vi "InstruDataRead_DP_ver2.1.vi"(8 "error in":errorcluster, 9 "memory of # of pts in buffer":i32[](array[numeric]), 10 "Const I output":dbl[](array[numeric]), 11 "output cluster":T1={"Main Sweep"=0, "Steps Config:"={"total points:"=0, "Step Delay (s)"=0.0, "Ini Delay (s)"=0.0, "# of steps:"=0}, "Temperature Control (ITC 503):"={"GPIB ADR"=0, "Change Heater?"={"Heater?"=FALSE, "Heater"=0}, "Change Temp?"={"Change T?"=FALSE, "Set T (K)"=0.0}, "Cluster"={"Heat Auto?"=FALSE, "Manual Heat?"=FALSE, "Heater (%)"=0.0}, "Change PID?"={"Change PID?"=FALSE, "P"=0.0, "I"=0.0, "D"=0.0}, "Change Para?"=FALSE, "Sensor"=1}, "Temperature Control (LS 340):"={"GPIB ADR"=0, "From (K)"=0.0, "To (K)"=0.0, "Rate (K/min)"=0.0, "Delta T (0.08K)"=0.0, "Temp. Header"="", "T Display Control"={"Ch B"=FALSE, "Ch C"=FALSE, "Ch D"=FALSE}}, "Magnet Control (IPS 120-10)"={"Action"=0, "Standby (s)"=0.0, "Heater on (s)"=0.0, "Sweep Setup "=[], "GPIB ADR"=0, "Change Para?"=FALSE}, "Keithley 6221 :"=[], "Measuring Instruments : "=[], "Lock-In SR7265 :"=[], "Deascription of \nthis measurement"="", "Instruments Config:"=[], "LS372 Bridge : 2"=[{"GPIB"=0, "Excitation"=0, "Autorange?"=FALSE, "Range"=0, "Current"=0, "Voltage"=0, "DataHeader"="Rx;Ry"}], "Magnet Control (CS4) 2"={"Action"=1, "Standby (s)"=0.0, "Heater on (s)"=300.0, "Sweep Setup "=[], "GPIB ADR"=0, "Change Para?"=FALSE}} {"Magnet Control (CS4) 2"."GPIB ADR" items=["None"=0, "25"=25]; "Magnet Control (CS4) 2"."Sweep Setup"."Rate in Range (T/min)" min=0.001 max=0.5 step=0.001; "Magnet Control (CS4) 2"."Sweep Setup"."Hold(min)" min=0.0; "Magnet Control (CS4) 2"."Sweep Setup"."Set Point (T)" min=-9.0 max=9.0 step=0.001; "Magnet Control (CS4) 2"."Action" items=["Up", "Down", "Pause", "Zero"]; "LS372 Bridge : 2"."Voltage" items=["2.00 uV"=1, "6.32 uV"=2, "20.0 uV"=3, "63.2 uV"=4, "200 uV"=5, "632 uV"=6, "2.0 mV"=7, "6.32 mV"=8]; "LS372 Bridge : 2"."Current" items=["1.00 pA"=1, "3.16 pA"=2, "10.0 pA"=3, "31.6 pA"=4, "100 pA"=5, "316 pA"=6, "1.00 nA"=7, "3.16 nA"=8, "10 nA"=9, "31.6 nA"=10, "100 nA"=11, "316 nA"=12, "1.00 uA"=13, "3.16 uA"=14, "10.0 uA"=15, "31.6 uA"=16, "100 uA"=17, "316 uA"=18, "1.00 mA"=19, "3.16 mA"=20, "10.0 mA"=21, "31.6 mA"=22]; "LS372 Bridge : 2"."Range" items=["2.0 m"=1, "6.32 m"=2, "20.0 m"=3, "63.2 m"=4, "200 m"=5, "632 m"=6, "2.00"=7, "6.32"=8, "20.0"=9, "63.2"=10, "200"=11, "632"=12, "2.00 k"=13, "6.32 k"=14, "20.0 k"=15, "63.2 k"=16, "200 k"=17, "632 k"=18, "2.00 M"=19, "6.32 M"=20, "20.0 M"=21, "63.2 M"=22]; "LS372 Bridge : 2"."Excitation" items=["Voltage", "Current"]; "LS372 Bridge : 2"."GPIB" items=["None"=0, "9"=9]; "Main Sweep" items=["Time", "DC Current", "Delta Current", "Pulse Delta Current", "Sine Current", "Lock-in Vosc"]; "Temperature Control (ITC 503):"."Sensor" items=["T2", "T3"]; "Magnet Control (IPS 120-10)"."Action" items=["Hold", "To Set point", "To Zero", "Clamp"]; "Keithley 6221 :"."Sweep Mode" items=["Linear", "Log", "Exp", "Inverse", "Manual"]}) -> (0 "error out":errorcluster, 1 "memory of # of pts in buffer update":i32[](array[numeric]), 2 "Data":dbl[](array[numeric]), 3 "output cluster 2":T1={"Main Sweep"=0, "Steps Config:"={"total points:"=0, "Step Delay (s)"=0.0, "Ini Delay (s)"=0.0, "# of steps:"=0}, "Temperature Control (ITC 503):"={"GPIB ADR"=0, "Change Heater?"={"Heater?"=FALSE, "Heater"=0}, "Change Temp?"={"Change T?"=FALSE, "Set T (K)"=0.0}, "Cluster"={"Heat Auto?"=FALSE, "Manual Heat?"=FALSE, "Heater (%)"=0.0}, "Change PID?"={"Change PID?"=FALSE, "P"=0.0, "I"=0.0, "D"=0.0}, "Change Para?"=FALSE, "Sensor"=1}, "Temperature Control (LS 340):"={"GPIB ADR"=0, "From (K)"=0.0, "To (K)"=0.0, "Rate (K/min)"=0.0, "Delta T (0.08K)"=0.0, "Temp. Header"="", "T Display Control"={"Ch B"=FALSE, "Ch C"=FALSE, "Ch D"=FALSE}}, "Magnet Control (IPS 120-10)"={"Action"=0, "Standby (s)"=0.0, "Heater on (s)"=0.0, "Sweep Setup "=[], "GPIB ADR"=0, "Change Para?"=FALSE}, "Keithley 6221 :"=[], "Measuring Instruments : "=[], "Lock-In SR7265 :"=[], "Deascription of \nthis measurement"="", "Instruments Config:"=[], "LS372 Bridge : 2"=[{"GPIB"=0, "Excitation"=0, "Autorange?"=FALSE, "Range"=0, "Current"=0, "Voltage"=0, "DataHeader"="Rx;Ry"}], "Magnet Control (CS4) 2"={"Action"=1, "Standby (s)"=0.0, "Heater on (s)"=300.0, "Sweep Setup "=[], "GPIB ADR"=0, "Change Para?"=FALSE}} {"Magnet Control (CS4) 2"."GPIB ADR" items=["None"=0, "25"=25]; "Magnet Control (CS4) 2"."Sweep Setup"."Rate in Range (T/min)" min=0.001 max=0.5 step=0.001; "Magnet Control (CS4) 2"."Sweep Setup"."Hold(min)" min=0.0; "Magnet Control (CS4) 2"."Sweep Setup"."Set Point (T)" min=-9.0 max=9.0 step=0.001; "Magnet Control (CS4) 2"."Action" items=["Up", "Down", "Pause", "Zero"]; "LS372 Bridge : 2"."Voltage" items=["2.00 uV"=1, "6.32 uV"=2, "20.0 uV"=3, "63.2 uV"=4, "200 uV"=5, "632 uV"=6, "2.0 mV"=7, "6.32 mV"=8]; "LS372 Bridge : 2"."Current" items=["1.00 pA"=1, "3.16 pA"=2, "10.0 pA"=3, "31.6 pA"=4, "100 pA"=5, "316 pA"=6, "1.00 nA"=7, "3.16 nA"=8, "10 nA"=9, "31.6 nA"=10, "100 nA"=11, "316 nA"=12, "1.00 uA"=13, "3.16 uA"=14, "10.0 uA"=15, "31.6 uA"=16, "100 uA"=17, "316 uA"=18, "1.00 mA"=19, "3.16 mA"=20, "10.0 mA"=21, "31.6 mA"=22]; "LS372 Bridge : 2"."Range" items=["2.0 m"=1, "6.32 m"=2, "20.0 m"=3, "63.2 m"=4, "200 m"=5, "632 m"=6, "2.00"=7, "6.32"=8, "20.0"=9, "63.2"=10, "200"=11, "632"=12, "2.00 k"=13, "6.32 k"=14, "20.0 k"=15, "63.2 k"=16, "200 k"=17, "632 k"=18, "2.00 M"=19, "6.32 M"=20, "20.0 M"=21, "63.2 M"=22]; "LS372 Bridge : 2"."Excitation" items=["Voltage", "Current"]; "LS372 Bridge : 2"."GPIB" items=["None"=0, "9"=9]; "Main Sweep" items=["Time", "DC Current", "Delta Current", "Pulse Delta Current", "Sine Current", "Lock-in Vosc"]; "Temperature Control (ITC 503):"."Sensor" items=["T2", "T3"]; "Magnet Control (IPS 120-10)"."Action" items=["Hold", "To Set point", "To Zero", "Clamp"]; "Keithley 6221 :"."Sweep Mode" items=["Linear", "Log", "Exp", "Inverse", "Manual"]}, 4 "B (T)":string, 5 "T2 (K)":string, 6 "T3 (K)":string, 7 "T1 (K)":string)   [LabVIEW 2012]
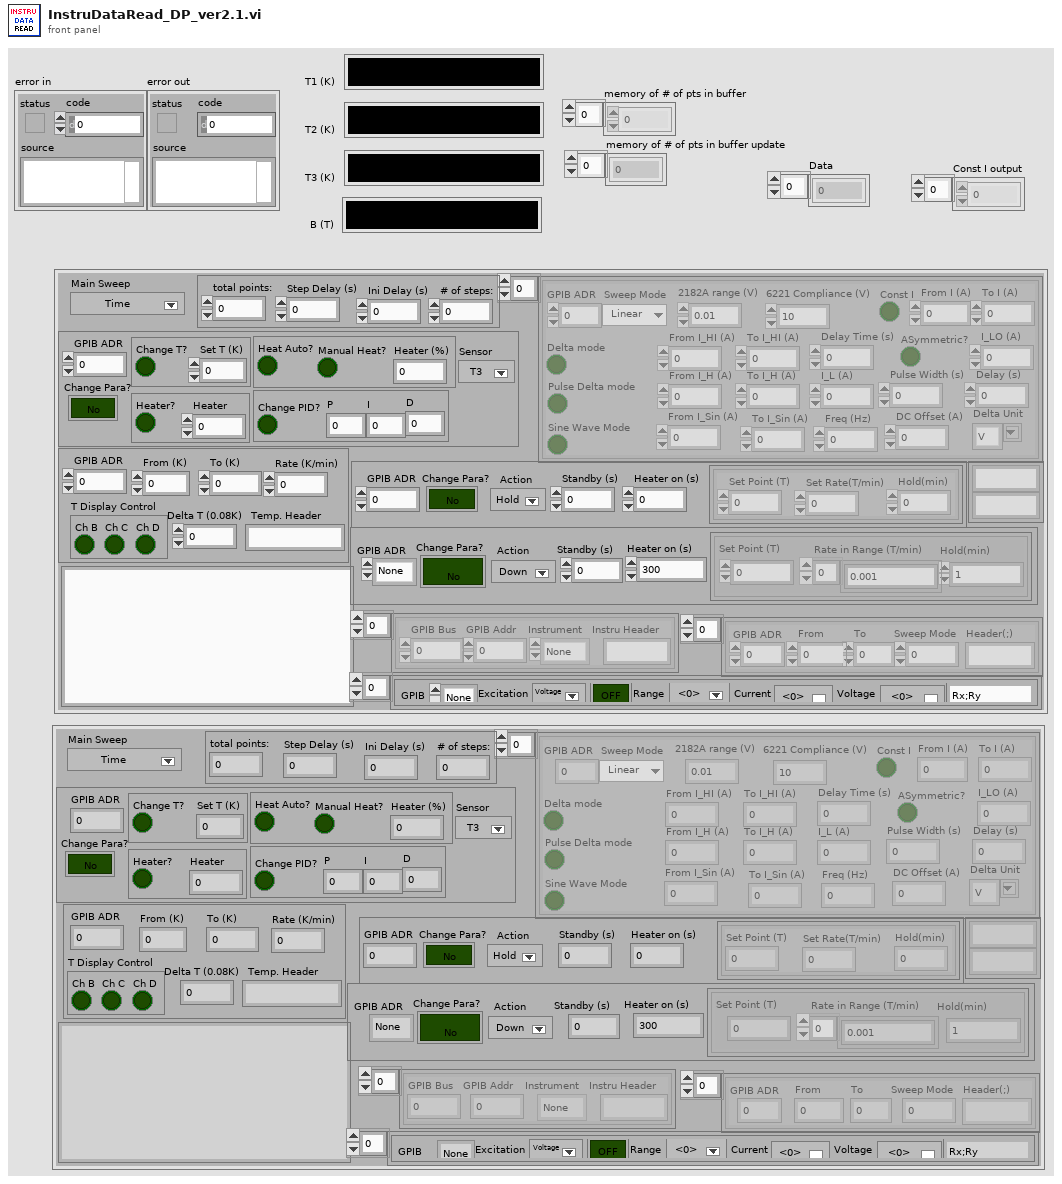
[diagram p1: front panel]
types:
  T1 = cluster{"Main Sweep":u8, "Steps Config:":cluster{"total points:":u32, "Step Delay (s)":dbl, "Ini Delay (s)":dbl, "# of steps:":u32}, "Temperature Control (ITC 503):":cluster{"GPIB ADR":u16, "Change Heater?":cluster{"Heater?":bool, "Heater":u8}, "Change Temp?":cluster{"Change T?":bool, "Set T (K)":dbl}, "Cluster":cluster{"Heat Auto?":bool, "Manual Heat?":bool, "Heater (%)":dbl}, "Change PID?":cluster{"Change PID?":bool, "P":dbl, "I":dbl, "D":dbl}, "Change Para?":bool, "Sensor":u16}, "Temperature Control (LS 340):":cluster{"GPIB ADR":u16, "From (K)":dbl, "To (K)":dbl, "Rate (K/min)":dbl, "Delta T (0.08K)":dbl, "Temp. Header":string, "T Display Control":cluster{"Ch B":bool, "Ch C":bool, "Ch D":bool}}, "Magnet Control (IPS 120-10)":cluster{"Action":u16, "Standby (s)":dbl, "Heater on (s)":dbl, "Sweep Setup ":cluster{"Set Point (T)":dbl, "Set Rate(T/min)":dbl, "Hold(min)":dbl}[], "GPIB ADR":u16, "Change Para?":bool}, "Keithley 6221 :":cluster{"Delta mode":bool, "Const I":bool, "Pulse Delta mode":bool, "Sine Wave Mode":bool, "From I_HI (A)":dbl, "From I (A)":dbl, "I_LO (A)":dbl, "From I_H (A)":dbl, "I_L (A)":dbl, "Freq (Hz)":dbl, "From I_Sin (A)":dbl, "DC Offset (A)":dbl, "Delay Time (s)":dbl, "Pulse Width (s)":dbl, "Delay (s)":dbl, "To I (A)":dbl, "ASymmetric?":bool, "To I_HI (A)":dbl, "To I_H (A)":dbl, "To I_Sin (A)":dbl, "GPIB ADR":u16, "Sweep Mode":u8, "Delta Unit":string, "2182A range (V)":dbl, "6221 Compliance (V)":dbl}[], "Measuring Instruments : ":cluster{"GPIB Bus":dbl, "GPIB Addr":dbl, "Instrument":enum16{"None", "HP34401DMM", "Lockin 7265", "HP3456/7A", "HP3478A", "HP3325FG", "Keithley2182A"}, "Instru Header":string}[], "Lock-In SR7265 :":cluster{"GPIB ADR":u16, "From":dbl, "To":dbl, "Header(;)":string, "Sweep Mode":u8}[], "Deascription of \nthis measurement":string, "Instruments Config:":string[][], "LS372 Bridge : 2":cluster{"GPIB":u16, "Excitation":u16, "Autorange?":bool, "Range":u16, "Current":u16, "Voltage":u16, "DataHeader":string}[], "Magnet Control (CS4) 2":cluster{"Action":u16, "Standby (s)":dbl, "Heater on (s)":dbl, "Sweep Setup ":cluster{"Set Point (T)":dbl, "Hold(min)":dbl, "Rate in Range (T/min)":dbl[]}[], "GPIB ADR":u16, "Change Para?":bool}}
  T2 = cluster{"GPIB":u16, "Excitation":u16, "Autorange?":bool, "Range":u16, "Current":u16, "Voltage":u16, "DataHeader":string}[]
  T3 = cluster{"Delta mode":bool, "Const I":bool, "Pulse Delta mode":bool, "Sine Wave Mode":bool, "From I_HI (A)":dbl, "From I (A)":dbl, "I_LO (A)":dbl, "From I_H (A)":dbl, "I_L (A)":dbl, "Freq (Hz)":dbl, "From I_Sin (A)":dbl, "DC Offset (A)":dbl, "Delay Time (s)":dbl, "Pulse Width (s)":dbl, "Delay (s)":dbl, "To I (A)":dbl, "ASymmetric?":bool, "To I_HI (A)":dbl, "To I_H (A)":dbl, "To I_Sin (A)":dbl, "GPIB ADR":u16, "Sweep Mode":u8, "Delta Unit":string, "2182A range (V)":dbl, "6221 Compliance (V)":dbl}[]
  T4 = cluster{"GPIB Bus":dbl, "GPIB Addr":dbl, "Instrument":enum16{"None", "HP34401DMM", "Lockin 7265", "HP3456/7A", "HP3478A", "HP3325FG", "Keithley2182A"}, "Instru Header":string}[]
  T5 = cluster{"GPIB ADR":u16, "From":dbl, "To":dbl, "Header(;)":string, "Sweep Mode":u8}[]
  T6 = enum16{"None", "HP34401DMM", "Lockin 7265", "HP3456/7A", "HP3478A", "HP3325FG"}
  T7 = enum16{"None", "HP34401DMM", "Lockin 7265", "HP3456/7A", "HP3478A", "HP3325FG", "Keithley2182A"}
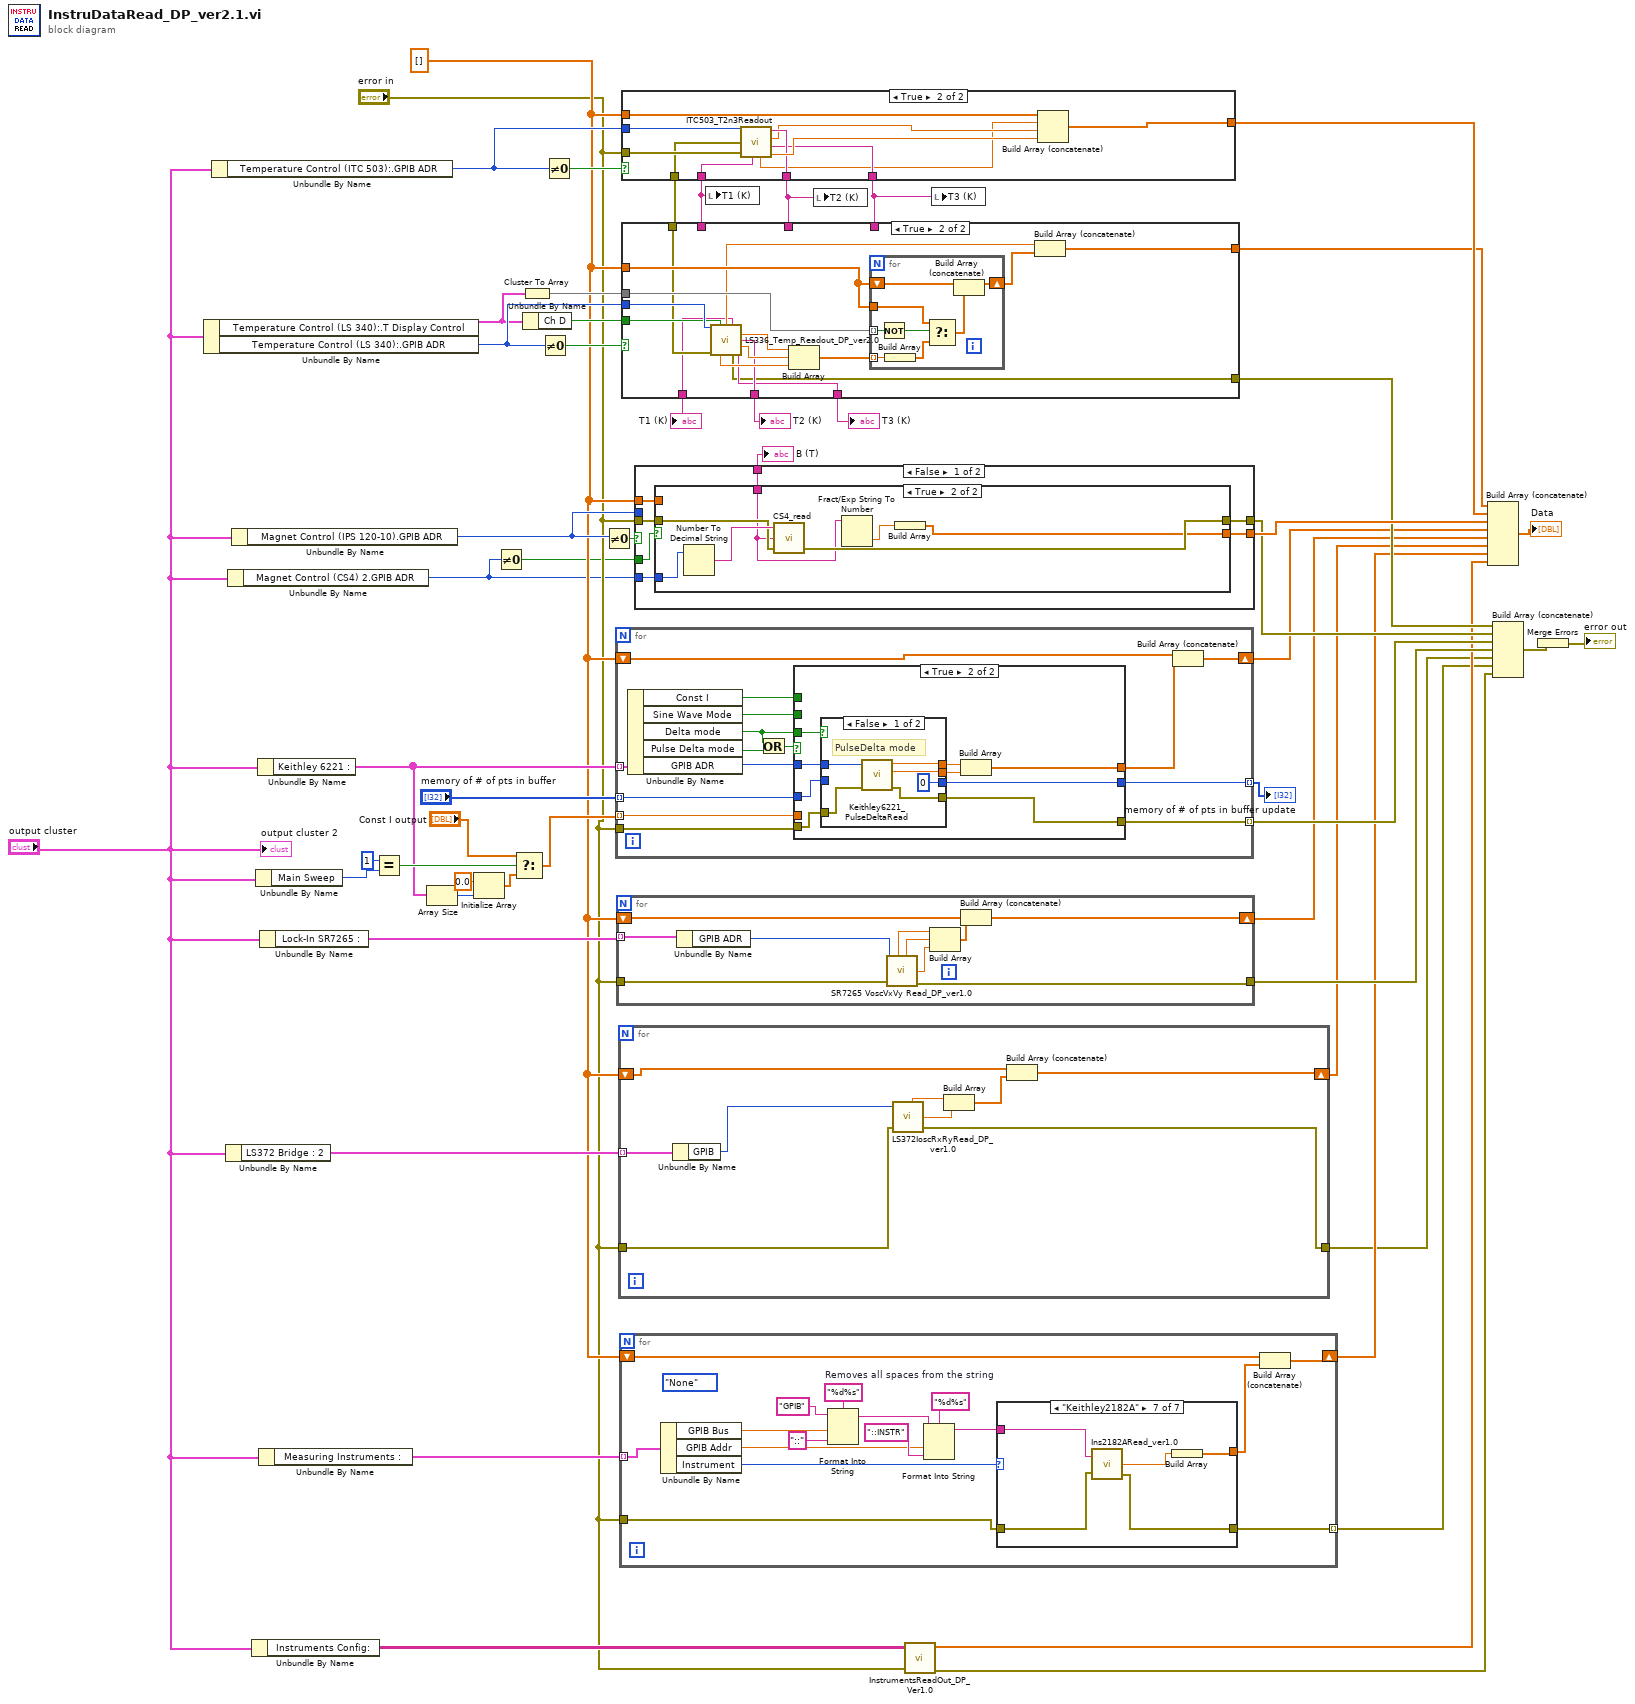
[diagram p0: block diagram]
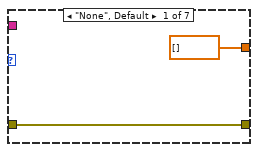
[diagram p2: hidden frame]
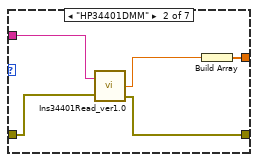
[diagram p3: hidden frame]
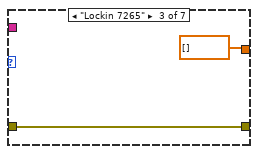
[diagram p4: hidden frame]
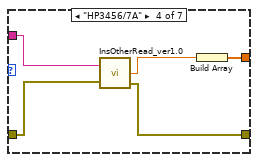
[diagram p5: hidden frame]
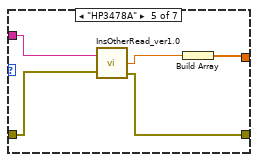
[diagram p6: hidden frame]
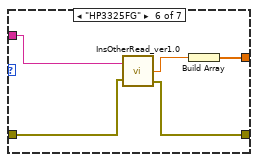
[diagram p7: hidden frame]
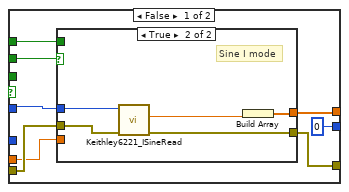
[diagram p8: hidden frame]
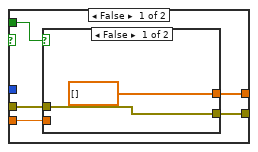
[diagram p9: hidden frame]
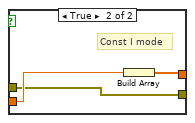
[diagram p10: hidden frame]
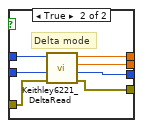
[diagram p11: hidden frame]
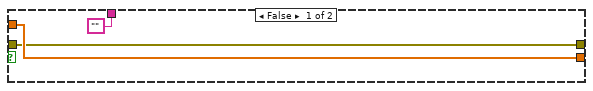
[diagram p12: hidden frame]
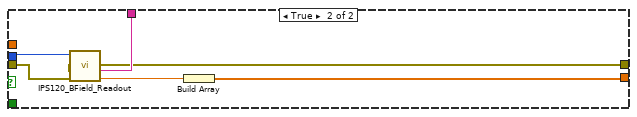
[diagram p13: hidden frame]
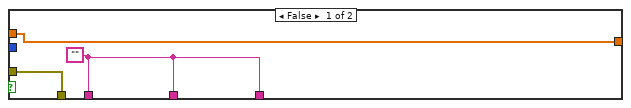
[diagram p14: hidden frame]
diagram:
  w7 = dbl[] []
  n1 = Unbundle By Name("output cluster") -> ("Temperature Control (LS 340):.T Display Control"=w52:cluster{"Ch B":bool, "Ch C":bool, "Ch D":bool}, "Temperature Control (LS 340):.GPIB ADR"=w54:u16)
  n2 = Unbundle By Name("output cluster") -> ("Temperature Control (ITC 503):.GPIB ADR"=w46:u16)
  n3 = Unbundle By Name("output cluster") -> ("LS372 Bridge : 2"=w8:T2)
  n4 = Unbundle By Name("output cluster") -> ("Magnet Control (CS4) 2.GPIB ADR"=w2:u16)
  n5 = Unbundle By Name("output cluster") -> ("Magnet Control (IPS 120-10).GPIB ADR"=w38:u16)
  n6 = Unbundle By Name("output cluster") -> ("Instruments Config:"=w26:string[][])
  n7 = Unbundle By Name("output cluster") -> ("Main Sweep"=w17:u8)
  n8 = Unbundle By Name("output cluster") -> ("Keithley 6221 :"=w12:T3)
  n9 = Unbundle By Name("output cluster") -> ("Measuring Instruments :"=w23:T4)
  n10 = Unbundle By Name("output cluster") -> ("Lock-In SR7265 :"=w29:T5)
  n11 = Equal?(x=u8 1, y=w17) -> (x = y?=w15:bool)
  n12 = Array Size(array=w12) -> (size(s)=w11:i32)
  n13 = Initialize Array(0.0 ("element"), w11) -> (w9:dbl[])
  n14 = Not Equal To 0?(x=w2) -> (x != 0?=w1:bool)
  n15 = Select(t="Const I output", s=w15, f=w9) -> (s? t:f=w14:dbl[])
  n16 = Cluster To Array(cluster=w52) -> (array=w51:bool[])
  n17 = Unbundle By Name(w52) -> ("Ch D"=w53:bool)
  n18 = Not Equal To 0?(x=w54) -> (x != 0?=w55:bool)
  n19 = Not Equal To 0?(x=w46) -> (x != 0?=w47:bool)
  n20 = Not Equal To 0?(x=w38) -> (x != 0?=w39:bool)
  n21 = for {
    tunnel: w12 -> [w70] mode=indexing
    tunnel: "error in" -> [w62]
    tunnel: [w61] -> w31 mode=indexing
    shift-right: [w60] -> w30
    shift-left: w7 -> [w68]
    tunnel: "memory of # of pts in buffer" -> [w59] mode=indexing
    tunnel: w14 -> [w57] mode=indexing
    tunnel: [w56] -> w18 mode=indexing
    n22 = Unbundle By Name(w70) -> ("Const I"=w58:bool, "Sine Wave Mode"=w63:bool, "Delta mode"=w65:bool, "Pulse Delta mode"=w67:bool, "GPIB ADR"=w69:u16)
    n23 = Or(x=w65, y=w67) -> (x .or. y?=w66:bool)
    n24 = case shown="True" w66 {
      tunnel: w69 -> [w77 w102]
      tunnel: w65 -> [_ w101]
      tunnel: [w78 w98] -> w64
      tunnel: w63 -> [w76 _]
      tunnel: w62 -> [w75 w97]
      tunnel: [w74 w96] -> w61
      tunnel: w59 -> [_ w95]
      tunnel: w58 -> [w73 _]
      tunnel: w57 -> [w72 _]
      tunnel: [0 ("memory of # of pts in buffer update") w94] -> w56
      frame False {
        n25 = case shown="True" w76 {
          tunnel: [w83 w93] -> w78
          tunnel: w77 -> [_ w91]
          tunnel: w75 -> [w82 w90]
          tunnel: [w81 w89] -> w74
          tunnel: w73 -> [w80 _]
          tunnel: w72 -> [w79 _]
          frame False {
            n26 = case shown="False" w80 {
              tunnel: [dbl[] [] w88] -> w83
              tunnel: w82 -> [w84 w86]
              tunnel: [w84 w86] -> w81
              tunnel: w79 -> [_ w87]
              frame False {
              }
              frame True {
                # "Const I mode"
                n27 = Build Array(w87) -> (w88:dbl[])
              }
            }
          }
          frame True {
            # "Sine I mode"
            n28 = call "Keithley6221_ISineRead.vi"("error in (no error)"=w90, "GPIB ADR"=w91) -> ("error out"=w89:errorcluster, "Reading"=w92:dbl)  [unwired: 7 in]
            n29 = Build Array(w92) -> (w93:dbl[])
          }
        }
      }
      frame True {
        n30 = case shown="False" w101 {
          tunnel: w102 -> [w108 w115]
          tunnel: [w107 w114] -> w99
          tunnel: [w106 w113] -> w100
          tunnel: w97 -> [w105 w112]
          tunnel: [w104 w111] -> w96
          tunnel: w95 -> [_ w110]
          tunnel: [0 ("memory of # of pts in buffer update") w109] -> w94
          frame False {
            # "PulseDelta mode"
            n31 = call "Keithley6221_PulseDeltaRead.vi"("error in (no error)"=w105, "GPIB ADR"=w108) -> ("error out"=w104:errorcluster, "Reading"=w107:dbl, "Pulse Delta Current High"=w106:dbl)  [unwired: 6 in]
          }
          frame True {
            # "Delta mode"
            n32 = call "Keithley6221_DeltaRead.vi"("error in (no error)"=w112, "memory of # of pts in buffer"=w110, "GPIB ADR"=w115) -> ("error out"=w111:errorcluster, "memory of # of pts in buffer update"=w109:i32, "Reading"=w114:dbl, "Delta Current High"=w113:dbl)  [unwired: 4 in]
          }
        }
        n33 = Build Array(w100, w99) -> (w98:dbl[])
      }
    }
    n34 = Build Array (concatenate)(w68, w64) -> (w60:dbl[])
  }
  "memory of # of pts in buffer update" <- w18
  n35 = for {
    shift-right: [w123] -> w28
    shift-left: w7 -> [w124]
    tunnel: "error in" -> [w122]
    tunnel: [w121] -> w27
    tunnel: w29 -> [w116] mode=indexing
    n36 = Unbundle By Name(w116) -> ("GPIB ADR"=w117:u16)
    n37 = call "SR7265 VoscVxVy Read_DP_ver1.0.vi"("GPIB ADR"=w117, "error in"=w122) -> ("Vosc (volt)"=w120:dbl, "Vx (volt)"=w119:dbl, "Vy (volt)"=w118:dbl, "error out"=w121:errorcluster)  [unwired: 3 in, 1 out]
    n38 = Build Array(w120, w119, w118) -> (w125:dbl[])
    n39 = Build Array (concatenate)(w124, w125) -> (w123:dbl[])
  }
  n40 = for {
    tunnel: w8 -> [w134] mode=indexing
    tunnel: "error in" -> [w127]
    shift-right: [w132] -> w5
    shift-left: w7 -> [w133]
    tunnel: [w126] -> w4
    n41 = Unbundle By Name(w134) -> ("GPIB"=w131:u16)
    n42 = call "LS372IoscRxRyRead_DP_ver1.0.vi"("GPIB ADR"=w131, "error in"=w127) -> ("Rx (Ohms)"=w130:dbl, "Ry (Ohms)"=w129:dbl, "error out"=w126:errorcluster)  [unwired: 4 in, 1 out]
    n43 = Build Array(w130, w129) -> (w128:dbl[])
    n44 = Build Array (concatenate)(w133, w128) -> (w132:dbl[])
  }
  n45 = for {
    tunnel: w23 -> [w150] mode=indexing
    tunnel: "error in" -> [w139]
    tunnel: [w138] -> w22 mode=indexing
    shift-right: [w136] -> w21
    shift-left: w7 -> [w137]
    w149 = "%d%s"  # Removes all spaces from the string
    (unwired) T6."None" ("Instrument")
    n46 = Unbundle By Name(w150) -> ("GPIB Bus"=w143:dbl, "GPIB Addr"=w142:dbl, "Instrument"=w141:T7)
    n47 = Format Into String(format string=w149, initial string="GPIB", w143, "::" ("input 2")) -> (resulting string=w146:string)  [unwired: 1 in, 1 out]
    n48 = Format Into String(format string="%d%s" ("Removes all labels from the string"), initial string=w146, w142, "::INSTR") -> (resulting string=w140:string)  [unwired: 1 in, 1 out]
    n49 = case shown="\"Keithley2182A\"" w141 {
      tunnel: w140 -> [_ w157 _ w164 w169 w174 w179]
      tunnel: w139 -> [w152 w155 w159 w162 w167 w171 w178]
      tunnel: [w152 w156 w159 w163 w168 w170 w177] -> w138
      tunnel: [dbl[] [] w154 dbl[] [] w160 w166 w172 w175] -> w135
      frame "None", Default {
      }
      frame "HP34401DMM" {
        n50 = call "Ins34401Read_ver1.0.vi"("VISA session"=w157, "error out"=w155) -> ("Numeric"=w153:dbl, "error out 2"=w156:errorcluster)  [unwired: 1 out]
        n51 = Build Array(w153) -> (w154:dbl[])
      }
      frame "Lockin 7265" {
      }
      frame "HP3456/7A" {
        n52 = call "InsOtherRead_ver1.0.vi"("VISA session"=w164, "error out"=w162) -> ("Numeric"=w161:dbl, "error out 2"=w163:errorcluster)  [unwired: 1 out]
        n53 = Build Array(w161) -> (w160:dbl[])
      }
      frame "HP3478A" {
        n54 = call "InsOtherRead_ver1.0.vi"("VISA session"=w169, "error out"=w167) -> ("Numeric"=w165:dbl, "error out 2"=w168:errorcluster)  [unwired: 1 out]
        n55 = Build Array(w165) -> (w166:dbl[])
      }
      frame "HP3325FG" {
        n56 = call "InsOtherRead_ver1.0.vi"("VISA session"=w174, "error out"=w171) -> ("Numeric"=w173:dbl, "error out 2"=w170:errorcluster)  [unwired: 1 out]
        n57 = Build Array(w173) -> (w172:dbl[])
      }
      frame "Keithley2182A" {
        n58 = call "Ins2182ARead_ver1.0.vi"("VISA session"=w179, "error out"=w178) -> ("Numeric"=w176:dbl, "error out 2"=w177:errorcluster)  [unwired: 1 out]
        n59 = Build Array(w176) -> (w175:dbl[])
      }
    }
    n60 = Build Array (concatenate)(w137, w135) -> (w136:dbl[])
  }
  n61 = case shown="True" w47 {
    tunnel: w46 -> [_ w193]
    tunnel: w7 -> [w180 w192]
    tunnel: [w180 w190] -> w41
    tunnel: "error in" -> [w181 w189]
    tunnel: [w181 w188] -> w45
    tunnel: [w182 w187] -> w44
    tunnel: [w182 w186] -> w43
    tunnel: [w182 w185] -> w42
    frame False {
      w182 = ""
    }
    frame True {
      n62 = call "ITC503_T2n3Readout.vi"("GPIB Address"=w193, "error in"=w189) -> ("error out"=w188:errorcluster, "Sensor T1"=w187:string, "Sensor T2"=w186:string, "T2"=w184:dbl, "T1"=w183:dbl, "Sensor T3"=w185:string, "T3"=w191:dbl)  [unwired: 2 out]
      n63 = Build Array (concatenate)(w192, w183, w184, w191) -> (w190:dbl[])
    }
  }
  n64 = case shown="True" w55 {
    tunnel: w54 -> [_ w214]
    tunnel: w53 -> [_ w213]
    tunnel: w7 -> [w198 w209]
    tunnel: w51 -> [_ w207]
    tunnel: [w198 w204] -> w40
    tunnel: w45 -> [w194 w203]
    tunnel: [w197 w202] -> w50
    tunnel: [w196 w201] -> w49
    tunnel: [w195 w200] -> w48
    tunnel: w44 -> [w197 _]
    tunnel: w43 -> [w196 _]
    tunnel: w42 -> [w195 _]
    tunnel: [w194 w199] -> w35
    frame False {
    }
    frame True {
      n65 = call "LS336_Temp_Readout_DP_ver2.0.vi"("GPIB ADR (18)"=w214, "Enable ChD (F)"=w213, "error in"=w203) -> (2:"Sensor A (K)"=w205:dbl, 3:"Sensor A (K)"=w202:string, 6:"Sensor B (K)"=w212:dbl, 8:"Sensor B (K)"=w201:string, 10:"Sensor C (K)"=w211:dbl, "Sensor D (K)"=w210:dbl, "error out"=w199:errorcluster, 15:"Sensor C (K)"=w200:string)  [unwired: 3 in, 2 out]
      n66 = Build Array(w212, w211, w210) -> (w208:dbl[])
      n67 = for {
        tunnel: w207 -> [w222] mode=indexing
        tunnel: w208 -> [w219] mode=indexing
        tunnel: w209 -> [w220]
        shift-right: [w216] -> w206
        shift-left: w209 -> [w217]
        n68 = Not(x=w222) -> (.not. x?=w221:bool)
        n69 = Build Array(w219) -> (w218:dbl[])
        n70 = Select(t=w220, s=w221, f=w218) -> (s? t:f=w215:dbl[])
        n71 = Build Array (concatenate)(w217, w215) -> (w216:dbl[])
      }
      n72 = Build Array (concatenate)(w205, w206) -> (w204:dbl[])
    }
  }
  "T1 (K)" <- w50
  "T2 (K)" <- w49
  "T3 (K)" <- w48
  n73 = case shown="False" w39 {
    tunnel: w38 -> [_ w245]
    tunnel: w7 -> [w228 _]
    tunnel: "error in" -> [w226 w244]
    tunnel: [w229 w243] -> w37
    tunnel: [w227 w241] -> w36
    tunnel: [w225 w240] -> w34
    tunnel: w2 -> [w223 _]
    tunnel: w1 -> [w224 _]
    frame False {
      n74 = case shown="True" w224 {
        tunnel: ["" w233] -> w229
        tunnel: w228 -> [w231 _]
        tunnel: [w231 w234] -> w227
        tunnel: w226 -> [w230 w237]
        tunnel: [w230 w236] -> w225
        tunnel: w223 -> [_ w239]
        frame False {
        }
        frame True {
          n75 = Number To Decimal String(number=w239) -> (decimal integer string=w238:string)  [unwired: 1 in]
          n76 = call "CS4_read.vi"("error in"=w237, "address string"=w238) -> ("error out"=w236:errorcluster, "Real Field"=w233:string)  [unwired: 2 out]
          n77 = Fract/Exp String To Number(string=w233) -> (number=w235:dbl)  [unwired: 3 in, 1 out]
          n78 = Build Array(w235) -> (w234:dbl[])
        }
      }
    }
    frame True {
      n79 = call "IPS120_BField_Readout.vi"("error in"=w244, "GPIB Address"=w245) -> (0:"B field read"=w242:dbl, 1:"B field read"=w243:string, "error out"=w240:errorcluster)  [unwired: 1 in, 2 out]
      n80 = Build Array(w242) -> (w241:dbl[])
    }
  }
  "B (T)" <- w37
  n81 = local write "T1 (K)"(w44) -> ()
  n82 = local write "T2 (K)"(w43) -> ()
  n83 = call "InstrumentsReadOut_DP_Ver1.0.vi"("Instruments Configs In 2D array"=w26, "error in"="error in") -> ("DataArray"=w25:dbl[], "error out"=w24:errorcluster)  [unwired: 4 in]
  n84 = local write "T3 (K)"(w42) -> ()
  n85 = Build Array (concatenate)(w40, w41, w36, w30, w28, w5, w21, w25) -> (→"Data":dbl[])
  n86 = Build Array (concatenate)(w35, w34, w31, w27, w4, w22, w24) -> (w33:errorcluster[])
  n87 = Merge Errors(w33) -> (→"error out":errorcluster)
  "output cluster 2" <- "output cluster"
